vi "Is king checked.vi"(8 "error in (no error)":errorcluster, 11 "Position in":refnum<class "Position.lvclass">) -> (0 "error out":errorcluster, 2 "King is checked":bool, 3 "Position out":refnum<class "Position.lvclass">)   [LabVIEW 2016, in "Chesslib.lvlib" / "Position.lvclass"]
uses:
  Position.lvclass
  Board/Board.lvclass
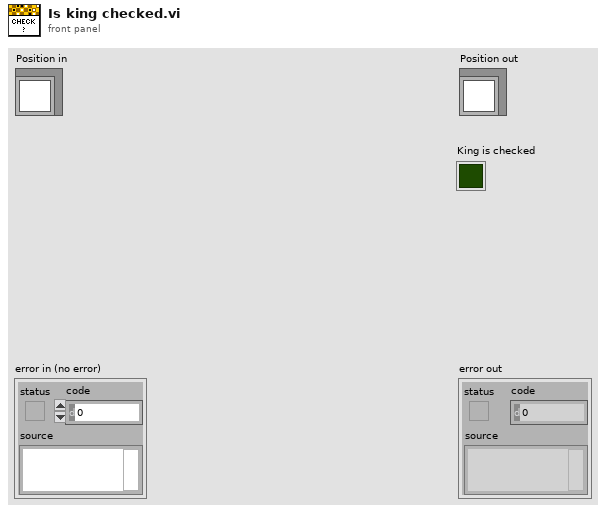
[diagram p1: front panel]
types:
  T1 = typedef "Chesslib.lvlib/Color.ctl" = enum16{"Light", "Dark"}
  T2 = typedef "Chesslib.lvlib/Square.ctl" = cluster{"File":T3, "Rank":T4}
  T3 = typedef "Chesslib.lvlib/File.ctl" = enum8{"a", "b", "c", "d", "e", "f", "g", "h"}
  T4 = typedef "Chesslib.lvlib/Rank.ctl" = enum8{"1", "2", "3", "4", "5", "6", "7", "8"}
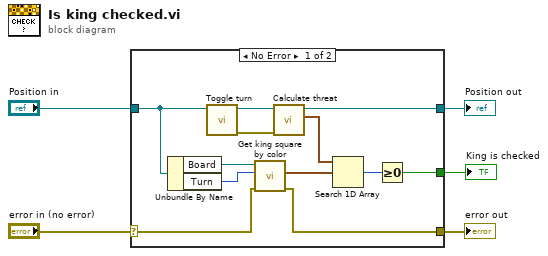
[diagram p0: block diagram]
diagram:
  n1 = case shown="No Error" "error in (no error)" {
    selector: "error in (no error)" -> [w8 w19]
    tunnel: [w7 w19] -> w4
    tunnel: [w16 w18] -> w2
    tunnel: "Position in" -> [w15 w18]
    tunnel: [w10 _] -> w1
    frame No Error {
      n2 = Unbundle By Name(w15) -> ("Board"=w14:refnum<class "Board.lvclass">, "Turn"=w13:T1)
      n3 = call "Toggle turn.vi"("Position in"=w15) -> ("error out"=w6:errorcluster, "Position out"=w17:refnum<class "Position.lvclass">)  [unwired: 9 in]
      n4 = call "Get king square by color.vi"("error in (no error)"=w8, "Color"=w13, "Board in"=w14) -> ("error out"=w7:errorcluster, "Square"=w9:T2)  [unwired: 5 in, 2 out]
      n5 = call "Calculate threat.vi"("error in (no error)"=w6, "Position in"=w17) -> ("Threatened squares"=w12:T2[], "Position out"=w16:refnum<class "Position.lvclass">)  [unwired: 7 in, 1 out]
      n6 = Search 1D Array(1D array=w12, element=w9) -> (index of element=w11:i32)  [unwired: 1 in]
      n7 = Greater Or Equal To 0?(x=w11) -> (x >= 0?=w10:bool)
    }
    frame Error {
    }
  }
  "error out" <- w4
  "Position out" <- w2
  "King is checked" <- w1
